vi "myRIO_BRig_RT_dataTrial_ENL2_time.vi"() -> (2 "output_ENL2_time":i32)   [LabVIEW 2014]
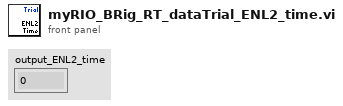
[diagram p1: front panel]
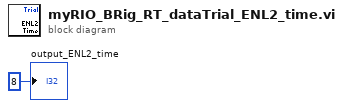
[diagram p0: block diagram]
diagram:
  "output_ENL2_time" <- 8 ("output_iBlock")
